vi "Encode Data.vi"(6 "numOfElements (1)":i32=1, 8 "offset":i32, 9 "dataType":string, 10 "Values Array in":dbl[](array[numeric]), 11 "changed flag array in":bool[](array[boolean])) -> (2 "raw data out":u8[](array[numeric]), 3 "changed flag array out":bool[](array[boolean]))   [LabVIEW 2019, in "HLA Custom Device Engine.lvlib"]
uses:
  HLA Custom Device Engine.lvlib
  Data Encoding_Decoding/HLA Data Conversion.lvlib
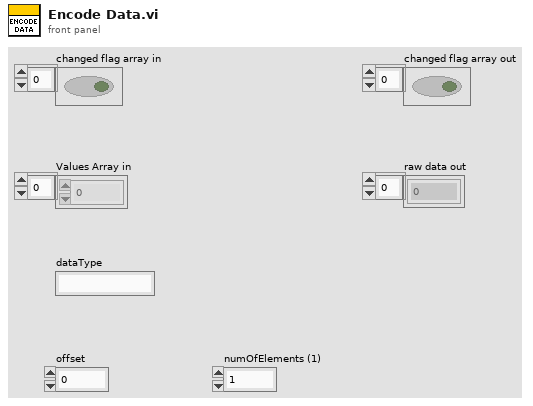
[diagram p1: front panel]
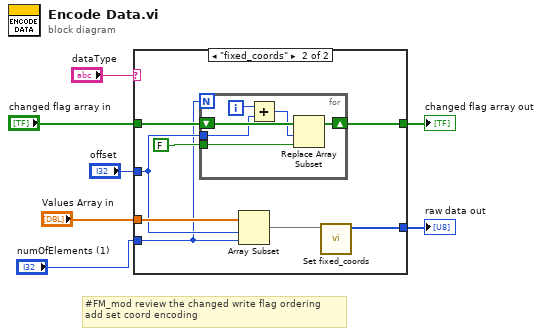
[diagram p0: block diagram]
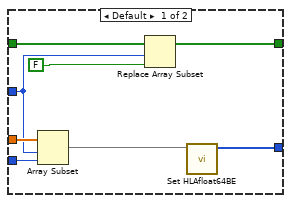
[diagram p2: hidden frame]
diagram:
  # "#FM_mod review the changed write flag ordering\nadd set coord encoding"
  n1 = case shown="\"fixed_coords\"" "dataType" {
    tunnel: "Values Array in" -> [w15 w23]
    tunnel: "offset" -> [w12 w21]
    tunnel: [w14 w16] -> w3
    tunnel: "changed flag array in" -> [w13 w22]
    tunnel: [w10 w19] -> w2
    tunnel: "numOfElements (1)" -> [w9 w18]
    frame Default {
      n2 = Array Subset(array=w15, index=w12, length=w9) -> (w8:dbl[])
      n3 = Replace Array Subset(array=w13, new element=FALSE ("new element/subarray"), index=w12) -> (w10:bool[])
      n4 = call "Set HLAfloat64BE.vi"("eu data in"=w8) -> ("raw data out"=w14:u8[])  [unwired: 9 in, 1 out]
    }
    frame "fixed_coords" {
      n5 = for {
        N: w18 -> [_]
        tunnel: w21 -> [w25]
        tunnel: FALSE ("new element/subarray") -> [w28]
        shift-right: [w27] -> w19
        shift-left: w22 -> [w29]
        i -> [w26]
        n6 = Add(x=w26, y=w25) -> (x+y=w24:i32)
        n7 = Replace Array Subset(array=w29, new element=w28, index=w24) -> (w27:bool[])
      }
      n8 = Array Subset(array=w23, index=w21, length=w18) -> (w17:dbl[])
      n9 = call "Set fixed_coords.vi"("eu data in"=w17) -> ("raw data out"=w16:u8[])  [unwired: 9 in, 1 out]
    }
  }
  "raw data out" <- w3
  "changed flag array out" <- w2
